vi "add.vi"(8 "error in (no error)":errorcluster, 11 "interfaceA in":refnum<class "interfaceA.lvclass">) -> (0 "error out":errorcluster, 3 "interfaceA out":refnum<class "interfaceA.lvclass">)   [LabVIEW 2020, in "interfaceA.lvclass"]
uses:
  interfaceA.lvclass
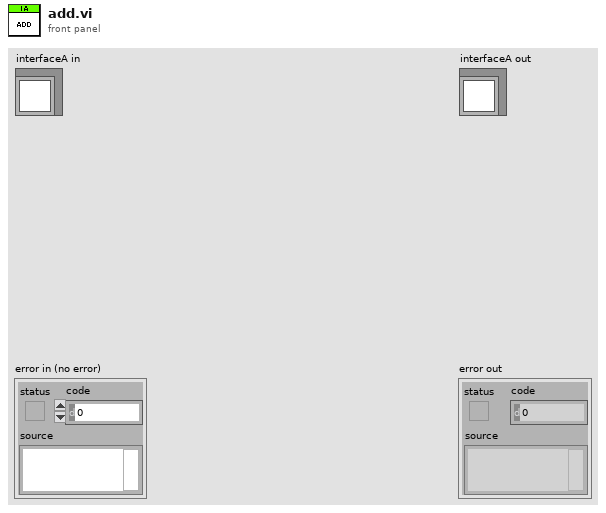
[diagram p1: front panel]
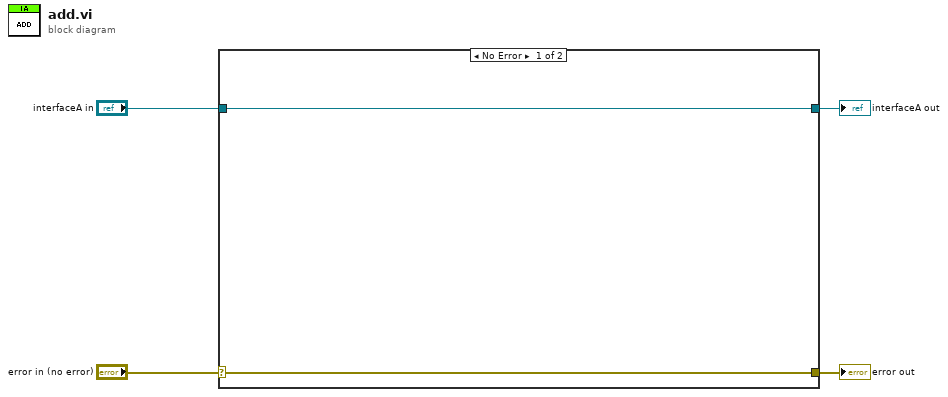
[diagram p0: block diagram]
diagram:
  n1 = case shown="No Error" "error in (no error)" {
    selector: "error in (no error)" -> [w5 w8]
    tunnel: [w5 w8] -> w3
    tunnel: [w6 w7] -> w1
    tunnel: "interfaceA in" -> [w6 w7]
    frame No Error {
    }
    frame Error {
    }
  }
  "error out" <- w3
  "interfaceA out" <- w1
